vi "RNN_proto.vi"(0 "seg_length":u64=2, 1 "dimension":u64=3, 3 "_hprev":T2=[[0.0], [0.0]], 5 "_params":T3={"Wxh"=[[0.578129, 2.569937, -0.0219857], [-2.46959, 0.027262, 2.449614362]], "Whh"=[[-1.3996, 0.961745], [0.364566, -0.477064]], "bh"=[[0.535351], [-1.985987]], "Why"=[[-0.658616, 0.764692], [-1.7789986, 0.388036], [-0.130912, -0.333988]], "by"=[[-0.528417], [-0.44032], [-0.8844819]]} {"Wxh" format="%_8f"; "Whh" format="%_8f"; "bh" format="%_8f"; "Why" format="%_8f"; "by" format="%_8f"}, 6 "Generate Sequences":bool, 7 "Seed Mode":enum16{"Random", "Fixed", "Continue", "Default"}(ring)=enum."Default", 8 "learning_rate":dbl=0.1, 9 "Fixed seed":u64, 11 "sample_length":u64=1, 12 "_sequence":u64[](array[numeric])=[1, 1, 1, 1], 13 "Learn/Sample":u64=1) -> (14 "xEntropy\n(Totals)":dbl[](array[numeric])=[4.019042439549509, 1.486931558997036] format="%_6f", 15 "Sequences Sampled":u64, 16 "xEntropy\n(Components)":dbl[][](array[numeric])=[[2.25897615466328, 1.7600662848862283], [1.486931558997036, 0.0]] format="%_6f", 17 "Sequences_":u64[][](array[numeric]), 21 "hs":dbl[][][](array[numeric]), 23 "h_latest":T2=[[0.7294195146201579], [-0.743695168691443]], 25 "params_":T3={"Wxh"=[[0.578129, 2.3699370053376954, -0.0219857], [-2.46959, 0.22726193094405095, 2.449614362]], "Whh"=[[-1.5995999892504944, 1.1617449510633957], [0.5645659922747992, -0.6770639469680022]], "bh"=[[0.33535100533769524], [-1.785987069055949]], "Why"=[[-0.658615999533275, 0.7646919998228623], [-1.5789986029136427, 0.18803600324004807], [-0.33091199882015726, -0.13398800114599535]], "by"=[[-0.5284169991570109], [-0.24032000191652825], [-1.084481899265759]]} {"Wxh" format="%_8f"; "Whh" format="%_8f"; "bh" format="%_8f"; "Why" format="%_8f"; "by" format="%_8f"})   [LabVIEW 2014]
uses:
  <vilib>/Analysis/Matrix/Datatypes/RealMatrix.ctl
  <vilib>/Analysis/Matrix/NI_Matrix.lvlib
panel:
  in  "?":T1(tab)
  out "Targets":u64[][](array[numeric])=[[1, 1], [1, 0]]
  out "dParams_":T4={"dWxh"=[[0.0, 0.33962128588539625, 0.0], [0.0, -0.296953463594456, 0.0]], "dWhh"=[[0.22667956392779695, -0.2362659091930602], [-0.27459968279372876, 0.22263645152462455]], "dbh"=[[0.33962128588539625], [-0.296953463594456]], "dWhy"=[[-0.3856903974871094, 0.4033716718902145], [-0.4326552137303272, 0.4063830524328116], [0.8183456112174368, -0.8097547243230261]], "dby"=[[-0.5457838548255013], [-0.5347967453478676], [1.080580600173369]]} {"dWxh" format="%_8f"; "dWhh" format="%_8f"; "dbh" format="%_8f"; "dWhy" format="%_8f"; "dby" format="%_8f"}
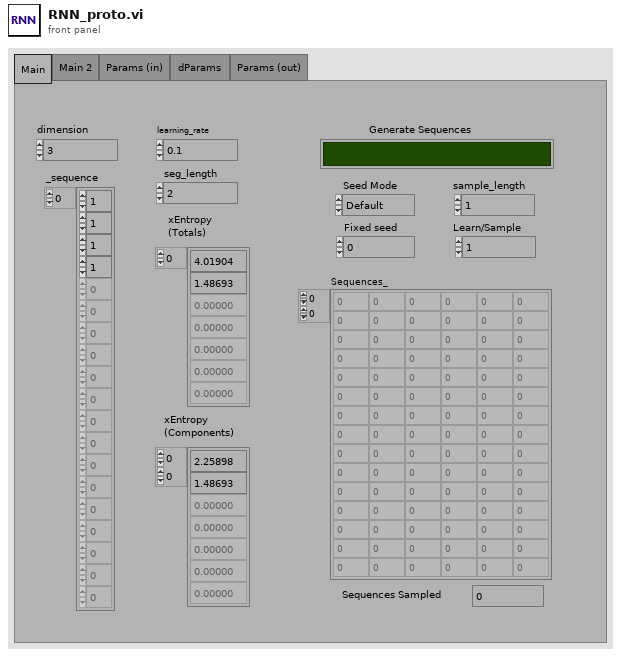
[diagram p1: front panel]
types:
  T1 = enum32{"Main", "Main 2", "Params (in)", "dParams ", "Params (out)"}
  T2 = typedef "NI_Matrix.lvlib/RealMatrix.ctl" = dbl[][]
  T3 = cluster{"Wxh":T2, "Whh":T2, "bh":T2, "Why":T2, "by":T2}
  T4 = cluster{"dWxh":T2, "dWhh":T2, "dbh":T2, "dWhy":T2, "dby":T2}
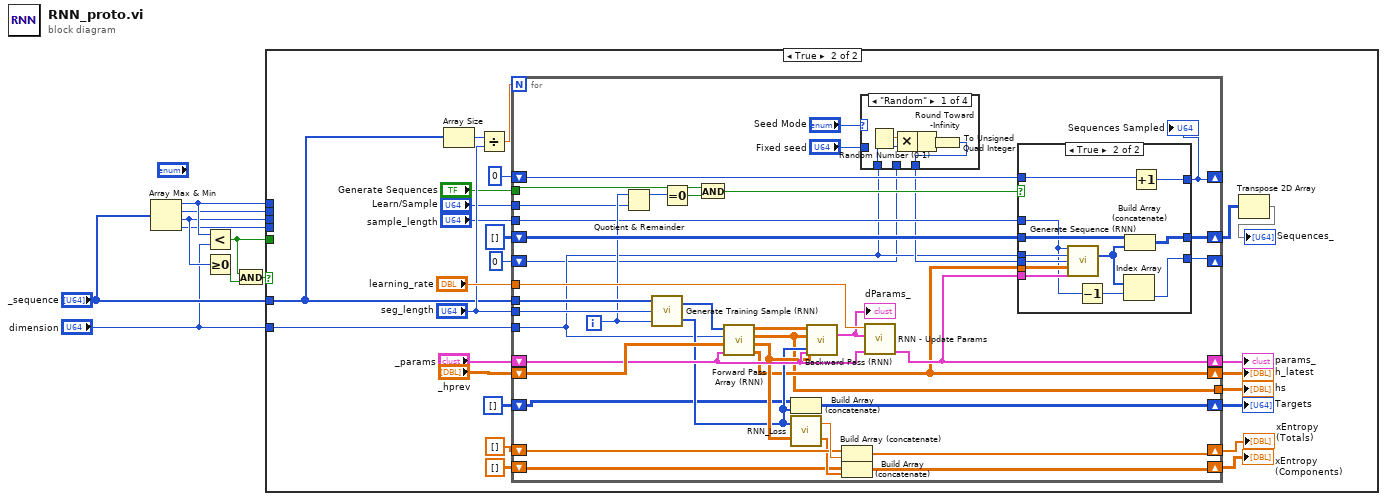
[diagram p0: block diagram]
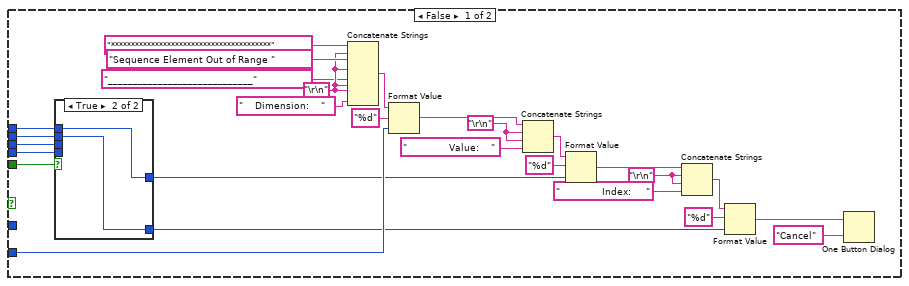
[diagram p2: hidden frame]
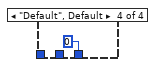
[diagram p6: hidden frame]
diagram:
  n1 = Array Max & Min(array="_sequence") -> (max value=w6:u64, max index (indices)=w5:i32, min value=w4:u64, min index (indices)=w3:i32)
  n2 = Less?(x=w6, y="dimension") -> (x < y?=w2:bool)
  n3 = Greater Or Equal To 0?(x=w4) -> (x >= 0?=w8:bool)
  n4 = And(x=w2, y=w8) -> (x .and. y?=w7:bool)
  n5 = case shown="True" w7 {
    tunnel: "_sequence" -> [_ w43]
    tunnel: "dimension" -> [w23 w42]
    tunnel: w6 -> [w31 _]
    tunnel: w5 -> [w30 _]
    tunnel: w4 -> [w29 _]
    tunnel: w3 -> [w28 _]
    tunnel: w2 -> [w27 _]
    frame False {
      w21 = "\r\n"
      w18 = "\r\n"
      w16 = "\r\n"
      n6 = case shown="True" w27 {
        tunnel: w31 -> [_ w40]
        tunnel: w30 -> [_ w39]
        tunnel: w29 -> [w38 _]
        tunnel: w28 -> [w37 _]
        tunnel: [w38 w40] -> w10
        tunnel: [w37 w39] -> w11
        frame False {
        }
        frame True {
        }
      }
      n7 = Concatenate Strings("****************************************" ("message"), w16, "Sequence Element Out of Range " ("message"), w16, "_____________________________" ("message"), w16, w16, "    Dimension:    " ("message")) -> (w35:string)
      n8 = Format Value(string ("")=w35, format string="%d", value (0)=w23) -> (output string=w19:string)
      n9 = Concatenate Strings(w19, w18, w18, "              Value:    " ("message")) -> (w32:string)
      n10 = Format Value(string ("")=w32, format string="%d", value (0)=w10) -> (output string=w20:string)
      n11 = Concatenate Strings(w20, w21, w21, "              Index:     " ("message")) -> (w25:string)
      n12 = Format Value(string ("")=w25, format string="%d", value (0)=w11) -> (output string=w24:string)
      n13 = One Button Dialog(message=w24, button name ("OK")="Cancel") -> ()  [unwired: 1 out]
    }
    frame True {
      n14 = Array Size(array=w43) -> (size(s)=w62:i32)
      n15 = Divide(x=w62, y="seg_length") -> (x/y=w63:dbl)
      n16 = for {
        N: w63 -> [_]
        tunnel: w43 -> [w98]
        tunnel: w42 -> [w68]
        tunnel: "learning_rate" -> [w101]
        shift-right: [w74] -> w53
        shift-left: "_hprev" -> [w102]
        shift-right: [w83] -> w54
        shift-left: "_params" -> [w100]
        tunnel: "seg_length" -> [w87]
        shift-right: [w95] -> w56
        shift-left: dbl[] [] -> [w94]
        shift-right: [w92] -> w55
        shift-left: dbl[][] [] -> [w91]
        shift-right: [w89] -> w57
        shift-left: u64[][] [] -> [w88]
        shift-right: [w85] -> w45
        shift-left: u64[][] [] -> [w86]
        tunnel: "Generate Sequences" -> [w77]
        shift-right: [w84] -> _
        shift-left: u64 0 ("Numeric") -> [w67]
        tunnel: "Learn/Sample" -> [w80]
        tunnel: "sample_length" -> [w75]
        shift-right: [w72] -> _
        shift-left: u64 0 ("Numeric") -> [w73]
        tunnel: [w66] -> w41
        i -> [w81]
        n17 = Quotient & Remainder(x=w81, y=w80) -> (x-y*floor(x/y)=w79:u64)  [unwired: 1 out]
        n18 = call "Generate Training Sample (RNN).vi"("iteration"=w81, "seg_length"=w87, "indices"=w98) -> ("targets"=w90:i64[], "inputs"=w97:i64[])
        n19 = Equal To 0?(x=w79) -> (x = 0?=w78:bool)
        n20 = And(x=w77, y=w78) -> (x .and. y?=w76:bool)
        n21 = call "Forward Pass Array (RNN).vi"("inputs"=w97, "dimension"=w68, "hprev"=w102, "params"=w100) -> ("xs"=w103:dbl[][][], "hs"=w66:dbl[][][], "ps"=w99:dbl[][][], "h_latest"=w74:T2)  [unwired: 3 in]
        n22 = Build Array (concatenate)(w88, w90) -> (w89:u64[][])
        n23 = call "RNN_Loss.vi"("targets"=w90, "ps"=w99) -> ("Loss (total)"=w96:dbl, "Loss Array"=w93:dbl[])  [unwired: 16 in]
        n24 = call "Backward Pass (RNN).vi"("xs"=w103, "hs"=w66, "ps"=w99, "targets"=w90, "params"=w100) -> ("dParams_"=w82:T4)  [unwired: 10 in]
        "dParams_" <- w82
        n25 = Build Array (concatenate)(w94, w96) -> (w95:dbl[])
        n26 = Build Array (concatenate)(w91, w93) -> (w92:dbl[][])
        n27 = case shown="\"Random\"" "Seed Mode" {
          tunnel: [w108 w109 w110 u64 0] -> w71
          tunnel: w68 -> [w107 _ _ _]
          tunnel: "Fixed seed" -> [_ w109 _ _]
          tunnel: w67 -> [_ _ w110 _]
          frame "Random" {
            n28 = Random Number (0-1)() -> (number: 0 to 1=w106:dbl)
            n29 = Multiply(x=w106, y=w107) -> (x*y=w105:dbl)
            n30 = Round Toward -Infinity(1:w105) -> (0:w104:dbl)
            n31 = To Unsigned Quad Integer(1:w104) -> (0:w108:u64)
          }
          frame "Fixed" {
          }
          frame "Continue" {
          }
          frame "Default", Default {
          }
        }
        n32 = call "RNN - Update Params.vi"("learning_rate"=w101, "dParams"=w82, "_params"=w100) -> ("params_"=w83:T3)  [unwired: 5 in]
        n33 = case shown="True" w76 {
          tunnel: w83 -> [_ w126]
          tunnel: w74 -> [_ w125]
          tunnel: w68 -> [_ w124]
          tunnel: w71 -> [w113 w123]
          tunnel: w86 -> [w114 w121]
          tunnel: [w114 w122] -> w85
          tunnel: [w113 w119] -> w84
          tunnel: w75 -> [_ w118]
          tunnel: [w112 w117] -> w72
          tunnel: w73 -> [w112 w116]
          frame False {
          }
          frame True {
            n34 = call "Generate Sequence (RNN).vi"("sample length"=w118, "dimension"=w124, "index seed"=w123, "hidden state (in)"=w125, "params"=w126) -> ("sequence out"=w120:u64[])  [unwired: 9 in, 1 out]
            n35 = Decrement(x=w118) -> (x-1=w115:u64)
            n36 = Index Array(array=w120, index=w115) -> (element=w119:u64)
            n37 = Build Array (concatenate)(w121, w120) -> (w122:u64[][])
            n38 = Increment(x=w116) -> (x+1=w117:u64)
          }
        }
        "Sequences Sampled" <- w72
      }
      "params_" <- w54
      "h_latest" <- w53
      "Targets" <- w57
      "xEntropy\n(Totals)" <- w56
      "xEntropy\n(Components)" <- w55
      "hs" <- w41
      n39 = Transpose 2D Array(2D array=w45) -> (transposed array=→"Sequences_":u64[][])
    }
  }
